vi "Edge or Level.vi"(8 "error in (no error)":errorcluster, 10 "Event types (Edge or Level)":u16(ring) items=["Edge", "Level"], 11 "VISA resource name":refnum<visa-resource-name>) -> (0 "error out":errorcluster, 3 "VISA resource name out":refnum<visa-resource-name>)   [LabVIEW 2017, in "Sefram DAS220.lvlib"]
doc: "Trigger using edge or level for simple channel and complex trigger types."
uses:
  <instrlib>/Sefram DAS220/Sefram DAS220.lvlib
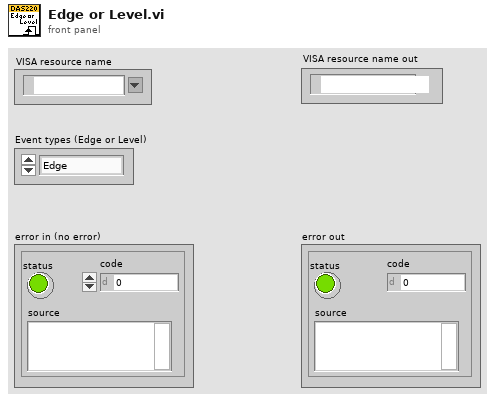
[diagram p1: front panel]
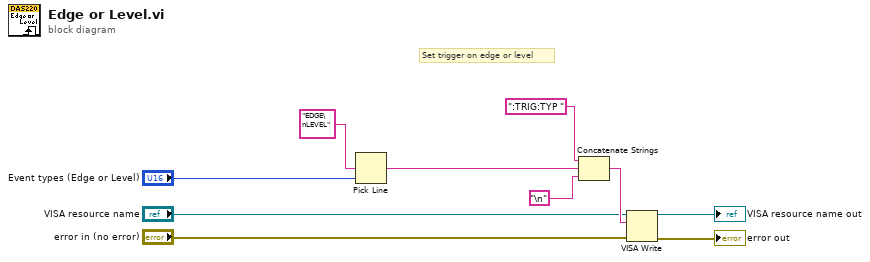
[diagram p0: block diagram]
diagram:
  # "Set trigger on edge or level"
  n1 = Pick Line(multi-line string="EDGE\nLEVEL", line index="Event types (Edge or Level)") -> (output string=w2:string)  [unwired: 1 in]
  n2 = Concatenate Strings(":TRIG:TYP " ("string"), w2, "\n") -> (w10:string)
  n3 = VISA Write(VISA resource name="VISA resource name", write buffer=w10, error in (no error)="error in (no error)") -> (VISA resource name out=→"VISA resource name out":refnum<visa-resource-name>, error out=→"error out":errorcluster)  [unwired: 1 out]
